vi "Send Reply Msg.vi"(7 "Message Priority (Normal)":T1=enum."Normal", 8 "error in":errorcluster, 9 "timeout in ms (-1)":i32=-1, 10 "Input":variant, 11 "Message Enqueuer":refnum<class "Message Enqueuer.lvclass">) -> (0 "error out":errorcluster, 1 "timed out?":bool, 2 "Reply":variant, 3 "Message Enqueuer out":refnum<class "Message Enqueuer.lvclass">)   [LabVIEW 2023, in "Target Reply Time Test Actor.lvlib" / "Reply Msg Msg.lvclass"]
doc: "This VI sends the message to an actor."
uses:
  Reply Msg Msg.lvclass
  <vilib>/ActorFramework/Message Enqueuer/Message Enqueuer.lvclass
  <vilib>/ActorFramework/Message Enqueuer/Message Priority.ctl
  C:/Program Files/National Instruments/LabVIEW 2023/vi.lib/ActorFramework/Reply Msg/Reply Msg.lvclass
  Reply Msg Msg.lvclass/Reply Msg Msg.ctl
  <vilib>/ActorFramework/Reply Msg/Reply Msg.lvclass/Reply Msg.ctl
  <vilib>/ActorFramework/Message Enqueuer/Message Enqueuer.lvclass/Message Enqueuer.ctl
  <vilib>/ActorFramework/Message Enqueuer/Enqueue.vi
  <vilib>/ActorFramework/Reply Msg/Reply Msg.lvclass
  C:/Program Files/National Instruments/LabVIEW 2023/vi.lib/ActorFramework/Message/Message.lvclass
  <vilib>/Utility/LVClass/Get LV Class Name.vi
  <resource>/AFDebug/Generate Trace for Message.vi
  <vilib>/ActorFramework/Message Priority Queue/Priority Enqueue.vi
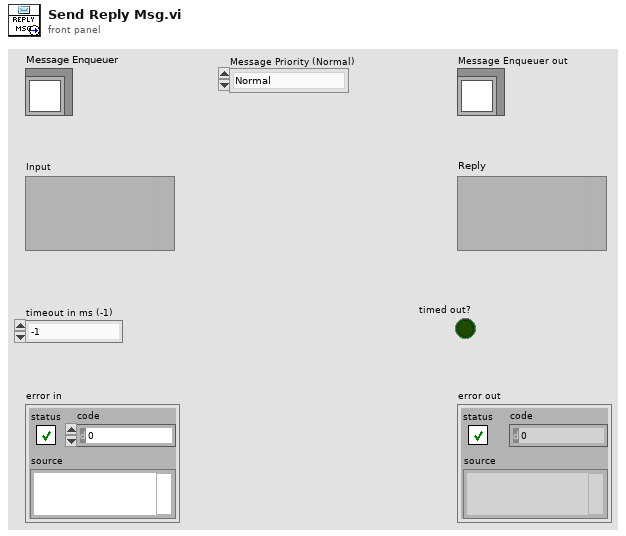
[diagram p1: front panel]
types:
  T1 = typedef "Actor Framework.lvlib/Message Enqueuer.lvclass/Message Priority.ctl" = enum16{"Low", "Normal", "High"}
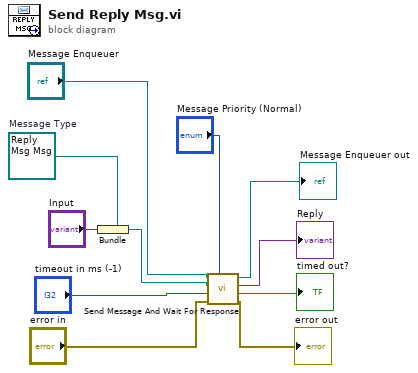
[diagram p0: block diagram]
diagram:
  w11 = refnum<class "Reply Msg Msg.lvclass"> refnum  # Message Type
  n1 = Bundle(cluster=w11, "Input") -> (w1:refnum<class "Reply Msg Msg.lvclass">)
  n2 = call <vilib>:"Send Message And Wait For Response.vi"("Message Priority (Normal)"="Message Priority (Normal)", "error in (no error)"="error in", "timeout in ms (-1)"="timeout in ms (-1)", "Original Message"=w1, "Message Enqueuer in"="Message Enqueuer") -> ("error out"=→"error out":errorcluster, "timed out?"=→"timed out?":bool, "Reply"=→"Reply":variant, "Message Enqueuer out"=→"Message Enqueuer out":refnum<class "Message Enqueuer.lvclass">)  [unwired: 3 in]
